vi "Configure Block Configuration List.vi"(6 "Index (1)":u32=1, 7 "Recall Operation (0: Next)":i32(ring) items=["Next", "Previous", "Recall"], 8 "error in (no error)":errorcluster, 9 "Configuration List (\"\")":string, 10 "Block Number (1)":u32=1, 11 "VISA resource name":refnum<visa-resource-name>) -> (0 "error out":errorcluster, 3 "VISA resource name out":refnum<visa-resource-name>)   [LabVIEW 2015, in "Keithley DMM6500 DAQ6500 Series.lvlib"]
doc: "Recalls, previous or next index of the settings at the configuration list."
uses:
  <instrlib>/Keithley DMM6500 DAQ6500 Series/Keithley DMM6500 DAQ6500 Series.lvlib
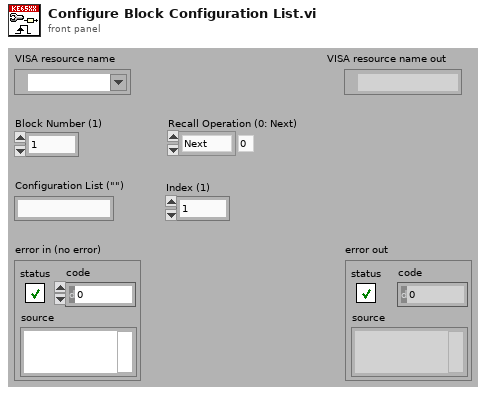
[diagram p1: front panel]
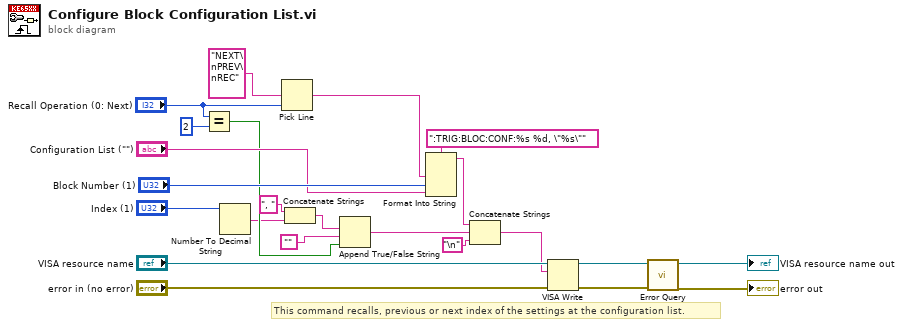
[diagram p0: block diagram]
diagram:
  # "This command recalls, previous or next index of the settings at the configuration list."
  n1 = Equal?(x="Recall Operation (0: Next)", y=2) -> (x = y?=w11:bool)
  n2 = Number To Decimal String(number="Index (1)") -> (decimal integer string=w3:string)  [unwired: 1 in]
  n3 = Pick Line(multi-line string="NEXT\nPREV\nREC", line index="Recall Operation (0: Next)") -> (output string=w15:string)  [unwired: 1 in]
  n4 = Concatenate Strings(", " ("string"), w3) -> (w4:string)
  n5 = Append True/False String(1:w11, 2:"", 3:w4) -> (0:w9:string)  [unwired: 1 in]
  n6 = Format Into String(format string=":TRIG:BLOC:CONF:%s %d, \"%s\"", w15, "Block Number (1)", "Configuration List (\"\")") -> (resulting string=w8:string)  [unwired: 2 in, 1 out]
  n7 = Concatenate Strings(w8, w9, "\n") -> (w7:string)
  n8 = VISA Write(VISA resource name="VISA resource name", write buffer=w7, error in (no error)="error in (no error)") -> (VISA resource name out=w20:refnum<visa-resource-name>, error out=w19:errorcluster)  [unwired: 1 out]
  n9 = call <instrlib>:"Error Query.vi"("error in (no error)"=w19, "VISA resource name"=w20) -> ("error out"=→"error out":errorcluster, "VISA resource name out"=→"VISA resource name out":refnum<visa-resource-name>)  [unwired: 6 in, 2 out]
